vi "EJEM9.vi"() -> ()   [LabVIEW 2013]
panel:
  in  "input 2":dbl
  in  "initial string 2":string
  out "concatenated string":string
  out "length":i32
  in  "string":string
  in  "input 1":dbl
  in  "initial string":string
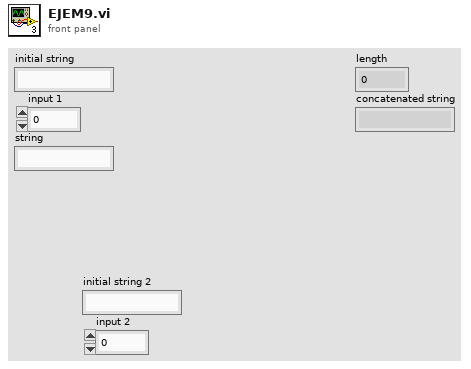
[diagram p1: front panel]
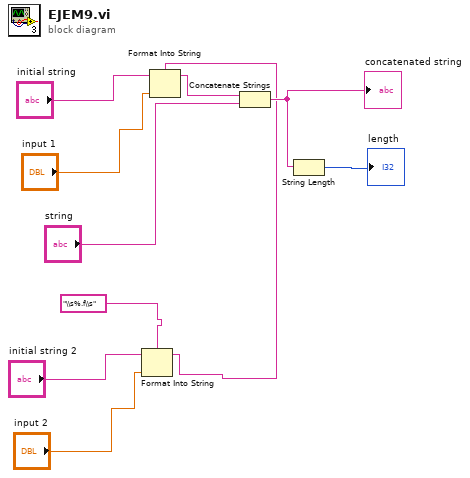
[diagram p0: block diagram]
diagram:
  n1 = Format Into String(format string="\\s%.f\\s", initial string="initial string 2", "input 2") -> (resulting string=w1:string)  [unwired: 1 in, 1 out]
  n2 = Format Into String(format string=w1, initial string="initial string", "input 1") -> (resulting string=w8:string)  [unwired: 1 in, 1 out]
  n3 = Concatenate Strings(w8, "string") -> (w6:string)
  "concatenated string" <- w6
  n4 = String Length(string=w6) -> (length=→"length":i32)
